vi "Send Raw Command.vi"(8 "error in (no error)":errorcluster, 10 "Raw Command":string, 11 "FW Arduino Control in":refnum<class "FW Arduino Control.lvclass">) -> (0 "error out":errorcluster, 3 "FW Arduino Control out":refnum<class "FW Arduino Control.lvclass">)   [LabVIEW 2024, in "FW Arduino Control.lvclass"]
uses:
  FW Arduino Control.lvclass
  Filter Wheel Object/Filter Wheel.lvclass
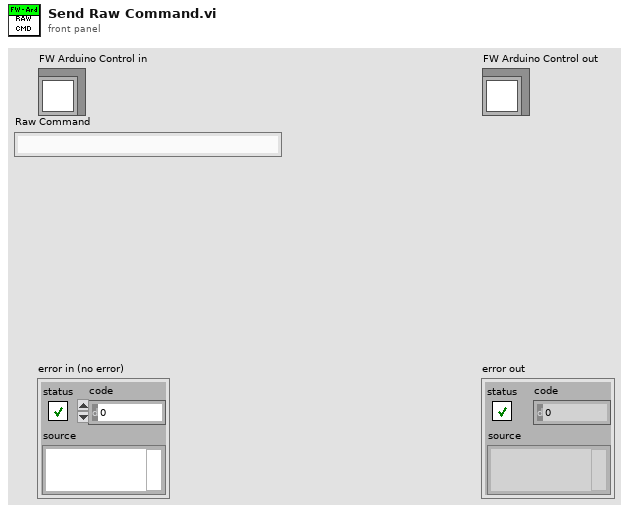
[diagram p1: front panel]
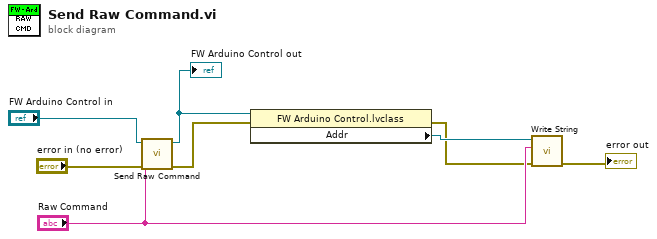
[diagram p0: block diagram]
diagram:
  n1 = call-parent "Send Raw Command.vi"("error in (no error)"="error in (no error)", "Raw Command"="Raw Command", "Filter Wheel in"="FW Arduino Control in") -> ("error out"=w3:errorcluster, "Filter Wheel out"=w6:refnum<class "FW Arduino Control.lvclass">)  [unwired: 7 in]
  "FW Arduino Control out" <- w6
  n2 = property class="FW Arduino Control.lvclass"(reference=w6, error in=w3) -> (error out=w2:errorcluster, "Addr"=w5:refnum<visa-resource-name>)  [unwired: 1 out]
  n3 = call "Write String.vi"("error in (no error)"=w2, "String"="Raw Command", "VISA resource name"=w5) -> ("error out"=→"error out":errorcluster)  [unwired: 7 in, 1 out]
